vi "AutoCal Password.vi"(7 "IonSniffer777":string="IonSniffer777") -> (1 "Advanced":bool, 3 "Valid":bool)   [LabVIEW 2015]
panel:
  in  "Remember My Password":bool
  in  "Password":string
  in  "Done":bool
  # "Please enter a valid password in order to access the selected feature.\n(note the password is case sensitive)"
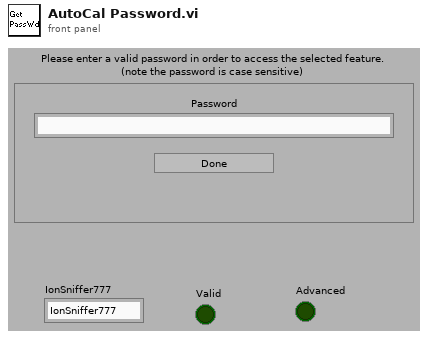
[diagram p1: front panel]
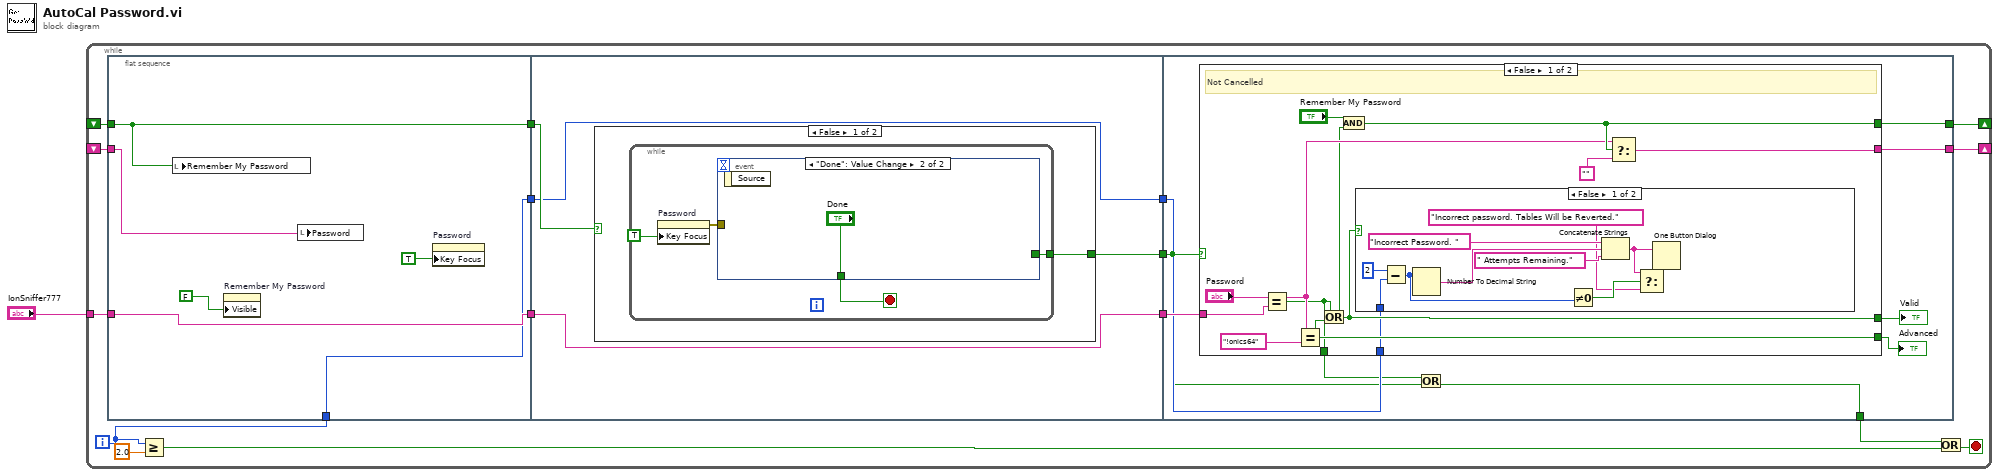
[diagram p0: block diagram]
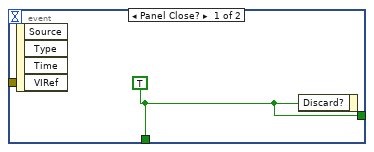
[diagram p2: hidden frame]
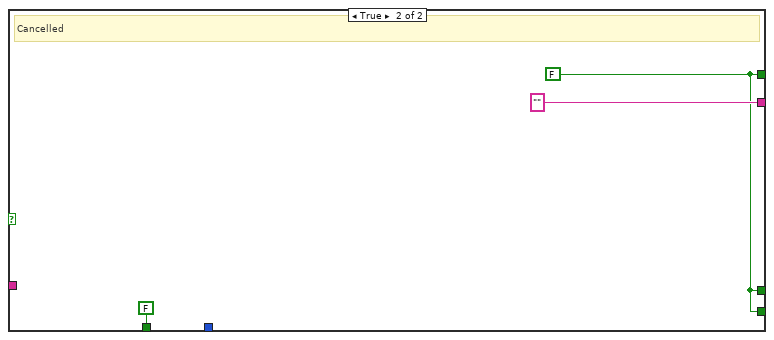
[diagram p5: hidden frame]
diagram:
  n1 = while {
    shift-right: [w17] -> _
    shift-left: _ -> [w16]
    shift-right: [w15] -> _
    shift-left: _ -> [w14]
    tunnel: "IonSniffer777" -> [w13]
    i -> [w8]
    stop <- w11 stop-if-true
    n2 = flat-sequence {
      tunnel: w16 -> [w22]
      tunnel: [w22] -> w7
      tunnel: w14 -> [w21]
      tunnel: w13 -> [w20]
      tunnel: [w20] -> w6
      tunnel: w8 -> [w19]
      tunnel: [w19] -> w5
      tunnel: w7 -> [w27]
      tunnel: w6 -> [w26]
      tunnel: [w26] -> w4
      tunnel: w5 -> [w25]
      tunnel: [w25] -> w3
      tunnel: [w24] -> w2
      tunnel: [w43] -> w17
      tunnel: [w42] -> w15
      tunnel: w4 -> [w41]
      tunnel: [w36] -> w12
      tunnel: w3 -> [w39]
      tunnel: w2 -> [w38]
      frame #0 {
        n3 = local write "Remember My Password"(w22) -> ()
        n4 = property on="Remember My Password" class="Bool (strict)"("Visible"=FALSE) -> ()  [unwired: 2 in, 2 out]
        n5 = local write "Password"(w21) -> ()
        n6 = property on="Password" class="Str"("Key Focus"=TRUE) -> ()  [unwired: 2 in, 2 out]
      }
      frame #1 {
        n7 = case shown="False" w27 {
          tunnel: [w28 _] -> w24
          frame False {
            n8 = while {
              tunnel: [w31] -> w28
              stop <- w32 stop-if-true
              n9 = property on="Password" class="Str"("Key Focus"=TRUE) -> (error out=w29:errorcluster)  [unwired: 2 in, 1 out]
              n10 = event shown="[1] \"Done\": Value Change" {
                selector: _ -> [_ _]
                dyn-events: _ -> [_ _]
                timeout: _ -> [_ _]
                tunnel: [w33 "Done"] -> w32
                tunnel: [w33 _] -> w31
                tunnel: w29 -> [_ _]
                event Panel Close? {
                  w33 = TRUE
                  n11 = event-data() -> ()  [unwired: 5 out]
                  n12 = event-data("Discard?"=w33) -> ()  [unwired: 1 in, 1 out]
                }
                event "Done": Value Change {
                  n13 = event-data() -> ()  [unwired: 2 out]
                }
              }
            }
          }
          frame True {
          }
        }
      }
      frame #2 {
        n14 = case shown="False" w38 {
          tunnel: [w53 w65] -> w43
          tunnel: [w51 "" ("Password")] -> w42
          tunnel: w41 -> [w50 _]
          tunnel: [w47 w65] -> w40
          tunnel: [w46 w65] -> w37
          tunnel: w39 -> [w45 _]
          tunnel: [w44 FALSE] -> w35
          frame False {
            # "Not Cancelled"
            n15 = Equal?(x="Password", y=w50) -> (x = y?=w44:bool)
            n16 = Equal?(x="Password", y="!onics64") -> (x = y?=w47:bool)
            n17 = Or(x=w44, y=w47) -> (x .or. y?=w46:bool)
            n18 = And(x="Remember My Password", y=w46) -> (x .and. y?=w53:bool)
            n19 = case shown="False" w46 {
              tunnel: w45 -> [w59 _]
              frame False {
                n20 = Subtract(x=2 ("y"), y=w59) -> (x-y=w56:i32)
                n21 = Number To Decimal String(number=w56) -> (decimal integer string=w61:string)  [unwired: 1 in]
                n22 = Not Equal To 0?(x=w56) -> (x != 0?=w58:bool)
                n23 = Concatenate Strings("Incorrect Password. " ("message"), w61, " Attempts Remaining." ("string")) -> (w55:string)
                n24 = Select(t=w55, s=w58, f="Incorrect password. Tables Will be Reverted.") -> ()  [unwired: 1 out]
                n25 = One Button Dialog(message=w55) -> ()  [unwired: 1 in, 1 out]
              }
              frame True {
              }
            }
            n26 = Select(t="Password", s=w53, f="") -> (s? t:f=w51:string)
          }
          frame True {
            w65 = FALSE
            # "Cancelled"
          }
        }
        "Valid" <- w37
        "Advanced" <- w40
        n27 = Or(x=w35, y=w38) -> (x .or. y?=w36:bool)
      }
    }
    n28 = Greater Or Equal?(x=w8, y=2.0) -> (x >= y?=w9:bool)
    n29 = Or(x=w12, y=w9) -> (x .or. y?=w11:bool)
  }
